vi "Dmm_menu_to_Dc_power.vi"(8 "error in (no error)":errorcluster, 11 "Measurement Type":T2(ring)) -> (0 "error out":errorcluster, 3 "output function":T1 items=["DC Voltage"=1006, "DC Current"=1007, "Pulse Voltage"=1049, "Pulse Current"=1050])   [LabVIEW 2021, in "niDCPower.lvclass"]
uses:
  niDCPower.lvclass
  <instrlib>/niDCPower/nidcpower.llb/niDCPower Output Function.ctl
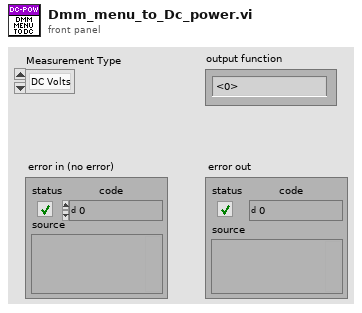
[diagram p1: front panel]
types:
  T1 = typedef "niDCPower Output Function.ctl" = i32
  T2 = enum32{"DC Volts", "AC Volts", "DC Current", "AC Current", "2-wire Resistance", "4-wire Resistance", "Diode", "Frequency", "Period", "AC Volts DC Coupled", "Capacitance", "Inductance", "Temperature"}
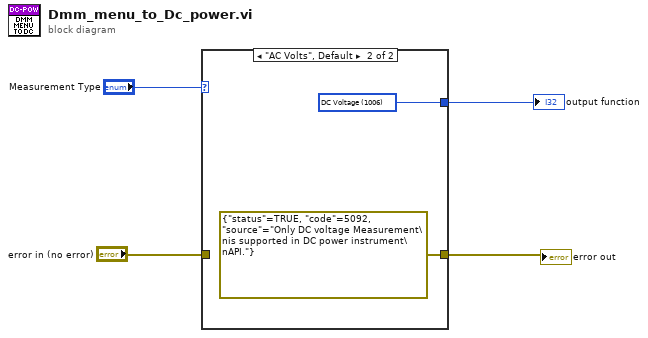
[diagram p0: block diagram]
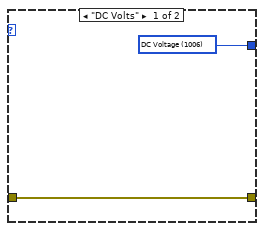
[diagram p2: hidden frame]
diagram:
  n1 = case shown="\"AC Volts\", Default" "Measurement Type" {
    tunnel: [w6 w8] -> w3
    tunnel: "error in (no error)" -> [w5 _]
    tunnel: [w5 errorcluster {"status"=TRUE, "code"=5092, "source"="Only DC voltage Measurement\nis supported in DC power instrument\nAPI."} ("error in (no error)")] -> w1
    frame "DC Volts" {
      w6 = T1 1006 items=["DC Voltage"=1006, "DC Current"=1007, "Pulse Voltage"=1049, "Pulse Current"=1050] ("output function")
    }
    frame "AC Volts", Default {
      w8 = T1 1006 items=["DC Voltage"=1006, "DC Current"=1007, "Pulse Voltage"=1049, "Pulse Current"=1050] ("output function")
    }
  }
  "output function" <- w3
  "error out" <- w1
